vi "OCV Histogram 4309.vi"(8 "Error In":errorcluster, 10 "Results Input":T2={"V ch0 Array"=[], "V ch1 Array"=[], "V ch2 Array"=[], "V ch3 Array"=[], "V ch4 Array"=[], "Elapsed Time (ms)"=11164, "DMM Fault Array"=[]}) -> (0 "Error Out":errorcluster, 1 "mean values of channels":dbl[](array[numeric])=[-6.648192609520545e-06, -2.6579412172609335e-06, 5.730660716698524e-06, 9.480335334891014e-06, -2.6031729589807576e-07] format="%#_7p", 2 "std dev":dbl=4.593584714427233e-07 format="%.3p", 3 "range":dbl=1.8604783993401584e-06 format="%.3p", 4 "Results Output":T1={"ch3 range"=1.5284304409643419e-06, "ch3 std dev"=3.7432297421944963e-07, "ch3 mean"=9.480335334891014e-06, "Histogram Graph ch3"={"X Values"=[8.804122636382775e-06, 8.956965680479209e-06, 9.109808724575643e-06, 9.262651768672077e-06, 9.415494812768511e-06, 9.568337856864946e-06, 9.72118090096138e-06, 9.874023945057814e-06, 1.0026866989154248e-05, 1.0179710033250682e-05], "Histogram: h(x)"=[2, 4, 3, 7, 5, 3, 7, 6, 1, 2]}, "ch2 range"=1.9041594218219493e-06, "ch2 std dev"=4.1579103732429095e-07, "ch2 mean"=5.730660716698524e-06, "Histogram Graph ch2"={"X Values"=[4.8417078226500296e-06, 5.032123764832224e-06, 5.222539707014419e-06, 5.412955649196613e-06, 5.603371591378808e-06, 5.7937875335610025e-06, 5.984203475743197e-06, 6.174619417925392e-06, 6.365035360107586e-06, 6.555451302289781e-06], "Histogram: h(x)"=[2, 2, 4, 3, 5, 8, 9, 5, 1, 1]}, "ch1 range"=1.7442902903444177e-06, "ch1 std dev"=4.468204660544414e-07, "ch1 mean"=-2.6579412172609335e-06, "Histogram Graph ch1"={"X Values"=[-3.3982864936427982e-06, -3.2238574646083565e-06, -3.0494284355739147e-06, -2.874999406539473e-06, -2.700570377505031e-06, -2.5261413484705894e-06, -2.3517123194361476e-06, -2.177283290401706e-06, -2.002854261367264e-06, -1.8284252323328223e-06], "Histogram: h(x)"=[4, 3, 5, 1, 6, 8, 4, 5, 3, 1]}, "ch0 range"=1.9838415017287296e-06, "ch0 std dev"=5.022029434534627e-07, "ch0 mean"=-6.648192609520545e-06, "Histogram Graph ch0"={"X Values"=[-7.4214795585101575e-06, -7.223095408337285e-06, -7.024711258164412e-06, -6.82632710799154e-06, -6.627942957818667e-06, -6.4295588076457944e-06, -6.231174657472922e-06, -6.032790507300049e-06, -5.8344063571271766e-06, -5.636022206954304e-06], "Histogram: h(x)"=[5, 3, 4, 6, 4, 8, 4, 1, 4, 1]}, "Waveform Chart ch1"=[-2.622437675041801e-06, -2.1054414953660847e-06, -2.3277676624794484e-06, -2.558376653803712e-06, -2.2236999675494533e-06, -2.589016451053761e-06, -2.6354278960691e-06, -2.7367192087189563e-06, -2.424017879995447e-06, -3.0489161443253215e-06, -3.1442148467963687e-06, -2.4032855210096374e-06, -2.569647882839888e-06, -2.4698150005498013e-06, -3.0781658817195746e-06, -2.377010372332436e-06, -2.0435595699758798e-06, -2.106839167327596e-06, -1.7412107178156014e-06, -3.2480049993772076e-06, -1.9805074376907754e-06, -2.5608807141114243e-06, -2.18054640635336e-06, -3.099457174386434e-06, -3.102303246629032e-06, -3.2920758007788295e-06, -3.3778499352142414e-06, -3.3187560901861313e-06, -3.484840052811922e-06, -3.485501008160019e-06, -2.8728971850629594e-06, -2.6623123946996634e-06, -2.187546597757112e-06, -2.5467930720162336e-06, -2.7862697099761513e-06, -2.528638777412977e-06, -2.0537236385737207e-06, -2.5329982714180255e-06, -2.7424337661967574e-06, -3.067742416854491e-06], "Waveform Chart ch2"=[5.544446756924017e-06, 5.893818847440082e-06, 5.6959361744068e-06, 6.353655436755351e-06, 6.650659273380882e-06, 6.187390686867271e-06, 6.20360970192913e-06, 5.7770612172558695e-06, 5.816303483036932e-06, 5.681492261411933e-06, 5.92762437831725e-06, 6.190843181120228e-06, 5.928079790707314e-06, 6.068116911256402e-06, 6.161619546592655e-06, 5.5543262999422065e-06, 6.17040032539053e-06, 5.4655577958543896e-06, 5.76704970728763e-06, 6.0194055222271105e-06, 5.783390336812049e-06, 5.768011867723238e-06, 6.0153044120154e-06, 6.001437704705948e-06, 5.911709913790112e-06, 5.830095407868431e-06, 5.25398022881523e-06, 5.15697143423068e-06, 4.826305970962092e-06, 5.462550730311096e-06, 5.059430867978049e-06, 5.682513029845579e-06, 5.851683523904261e-06, 5.099226732675129e-06, 5.2309820281174504e-06, 5.22374278950658e-06, 5.829274618675769e-06, 4.746499851558932e-06, 5.396447289671177e-06, 6.039472630669777e-06], "Waveform Chart ch0"=[-6.482741875349764e-06, -6.609674165618734e-06, -6.233203080218623e-06, -6.613210951394088e-06, -5.909245924550351e-06, -6.1328996888307884e-06, -6.358200673203053e-06, -6.870973185430456e-06, -6.243427483099904e-06, -5.953840097279857e-06, -6.577614794730629e-06, -5.768388563769013e-06, -5.889962020259323e-06, -5.91212430154465e-06, -6.419565311385181e-06, -6.50829315132552e-06, -5.536830131867864e-06, -6.271011369459595e-06, -6.937542782195293e-06, -7.44168991871554e-06, -6.8984467501811205e-06, -7.4441074466820366e-06, -6.884514522294152e-06, -7.229455884586274e-06, -7.204633996616539e-06, -7.520671633596594e-06, -7.348344858091178e-06, -7.026224856705287e-06, -6.4957495291395714e-06, -6.9697185324009035e-06, -6.64170832689038e-06, -6.516226556717238e-06, -6.80187883727134e-06, -7.473746530800666e-06, -6.8019074543289836e-06, -6.421730747707948e-06, -6.915517716049444e-06, -7.233306065769019e-06, -6.9335647318597554e-06, -6.495809932905111e-06], "Waveform Chart ch3"=[9.329772359568193e-06, 9.772186603754015e-06, 9.974785258468733e-06, 1.02561315552989e-05, 9.495402230894659e-06, 9.736598828932665e-06, 9.898850155608759e-06, 1.0197036488504313e-05, 9.305987891150035e-06, 9.316802834906767e-06, 9.746712874470878e-06, 9.737416581604666e-06, 9.867514527065477e-06, 9.509080464808271e-06, 9.481845866845764e-06, 9.70755176396829e-06, 8.885838770613302e-06, 9.475699672125386e-06, 9.258180372816345e-06, 9.834891872602234e-06, 9.402243918552161e-06, 9.713205786936326e-06, 9.876491292911543e-06, 9.871789580104262e-06, 9.650930388911628e-06, 9.41118365911455e-06, 9.575353492249282e-06, 9.196921234035763e-06, 9.15123272945548e-06, 8.949563027841687e-06, 9.474861956745276e-06, 8.825224921180636e-06, 8.727701114334558e-06, 9.16860173648142e-06, 8.905227736485157e-06, 9.144446889757383e-06, 8.885482293855075e-06, 9.859395612279415e-06, 9.32444154185109e-06, 9.310827508550253e-06]} {"ch3 range" format="%#_6p"; "ch3 std dev" format="%#.3p"; "ch3 mean" format="%#.6p"; "ch2 range" format="%#_6p"; "ch2 std dev" format="%#.3p"; "ch2 mean" format="%#.6p"; "ch1 range" format="%#_6p"; "ch1 std dev" format="%#.3p"; "ch1 mean" format="%#.6p"; "ch0 range" format="%#_6p"; "ch0 std dev" format="%#.3p"; "ch0 mean" format="%#.6p"}, 5 "Elapsed Time (ms)":u32)   [LabVIEW 2019]
uses:
  OCVResults.ctl
  Chart_Graph_Mean_Range_StdDev.ctl
  <vilib>/Analysis/baseanly.llb/Mean (DBL).vi
  <vilib>/Analysis/NI_AALBase.lvlib
  <vilib>/gmath/NI_Gmath.lvlib
panel:
  in  "Results Cluster":T1={"ch3 range"=1.5284304409643419e-06, "ch3 std dev"=3.7432297421944963e-07, "ch3 mean"=9.480335334891014e-06, "Histogram Graph ch3"={"X Values"=[8.804122636382775e-06, 8.956965680479209e-06, 9.109808724575643e-06, 9.262651768672077e-06, 9.415494812768511e-06, 9.568337856864946e-06, 9.72118090096138e-06, 9.874023945057814e-06, 1.0026866989154248e-05, 1.0179710033250682e-05], "Histogram: h(x)"=[2, 4, 3, 7, 5, 3, 7, 6, 1, 2]}, "ch2 range"=1.9041594218219493e-06, "ch2 std dev"=4.1579103732429095e-07, "ch2 mean"=5.730660716698524e-06, "Histogram Graph ch2"={"X Values"=[4.8417078226500296e-06, 5.032123764832224e-06, 5.222539707014419e-06, 5.412955649196613e-06, 5.603371591378808e-06, 5.7937875335610025e-06, 5.984203475743197e-06, 6.174619417925392e-06, 6.365035360107586e-06, 6.555451302289781e-06], "Histogram: h(x)"=[2, 2, 4, 3, 5, 8, 9, 5, 1, 1]}, "ch1 range"=1.7442902903444177e-06, "ch1 std dev"=4.468204660544414e-07, "ch1 mean"=-2.6579412172609335e-06, "Histogram Graph ch1"={"X Values"=[-3.3982864936427982e-06, -3.2238574646083565e-06, -3.0494284355739147e-06, -2.874999406539473e-06, -2.700570377505031e-06, -2.5261413484705894e-06, -2.3517123194361476e-06, -2.177283290401706e-06, -2.002854261367264e-06, -1.8284252323328223e-06], "Histogram: h(x)"=[4, 3, 5, 1, 6, 8, 4, 5, 3, 1]}, "ch0 range"=1.9838415017287296e-06, "ch0 std dev"=5.022029434534627e-07, "ch0 mean"=-6.648192609520545e-06, "Histogram Graph ch0"={"X Values"=[-7.4214795585101575e-06, -7.223095408337285e-06, -7.024711258164412e-06, -6.82632710799154e-06, -6.627942957818667e-06, -6.4295588076457944e-06, -6.231174657472922e-06, -6.032790507300049e-06, -5.8344063571271766e-06, -5.636022206954304e-06], "Histogram: h(x)"=[5, 3, 4, 6, 4, 8, 4, 1, 4, 1]}, "Waveform Chart ch1"=[-2.622437675041801e-06, -2.1054414953660847e-06, -2.3277676624794484e-06, -2.558376653803712e-06, -2.2236999675494533e-06, -2.589016451053761e-06, -2.6354278960691e-06, -2.7367192087189563e-06, -2.424017879995447e-06, -3.0489161443253215e-06, -3.1442148467963687e-06, -2.4032855210096374e-06, -2.569647882839888e-06, -2.4698150005498013e-06, -3.0781658817195746e-06, -2.377010372332436e-06, -2.0435595699758798e-06, -2.106839167327596e-06, -1.7412107178156014e-06, -3.2480049993772076e-06, -1.9805074376907754e-06, -2.5608807141114243e-06, -2.18054640635336e-06, -3.099457174386434e-06, -3.102303246629032e-06, -3.2920758007788295e-06, -3.3778499352142414e-06, -3.3187560901861313e-06, -3.484840052811922e-06, -3.485501008160019e-06, -2.8728971850629594e-06, -2.6623123946996634e-06, -2.187546597757112e-06, -2.5467930720162336e-06, -2.7862697099761513e-06, -2.528638777412977e-06, -2.0537236385737207e-06, -2.5329982714180255e-06, -2.7424337661967574e-06, -3.067742416854491e-06], "Waveform Chart ch2"=[5.544446756924017e-06, 5.893818847440082e-06, 5.6959361744068e-06, 6.353655436755351e-06, 6.650659273380882e-06, 6.187390686867271e-06, 6.20360970192913e-06, 5.7770612172558695e-06, 5.816303483036932e-06, 5.681492261411933e-06, 5.92762437831725e-06, 6.190843181120228e-06, 5.928079790707314e-06, 6.068116911256402e-06, 6.161619546592655e-06, 5.5543262999422065e-06, 6.17040032539053e-06, 5.4655577958543896e-06, 5.76704970728763e-06, 6.0194055222271105e-06, 5.783390336812049e-06, 5.768011867723238e-06, 6.0153044120154e-06, 6.001437704705948e-06, 5.911709913790112e-06, 5.830095407868431e-06, 5.25398022881523e-06, 5.15697143423068e-06, 4.826305970962092e-06, 5.462550730311096e-06, 5.059430867978049e-06, 5.682513029845579e-06, 5.851683523904261e-06, 5.099226732675129e-06, 5.2309820281174504e-06, 5.22374278950658e-06, 5.829274618675769e-06, 4.746499851558932e-06, 5.396447289671177e-06, 6.039472630669777e-06], "Waveform Chart ch0"=[-6.482741875349764e-06, -6.609674165618734e-06, -6.233203080218623e-06, -6.613210951394088e-06, -5.909245924550351e-06, -6.1328996888307884e-06, -6.358200673203053e-06, -6.870973185430456e-06, -6.243427483099904e-06, -5.953840097279857e-06, -6.577614794730629e-06, -5.768388563769013e-06, -5.889962020259323e-06, -5.91212430154465e-06, -6.419565311385181e-06, -6.50829315132552e-06, -5.536830131867864e-06, -6.271011369459595e-06, -6.937542782195293e-06, -7.44168991871554e-06, -6.8984467501811205e-06, -7.4441074466820366e-06, -6.884514522294152e-06, -7.229455884586274e-06, -7.204633996616539e-06, -7.520671633596594e-06, -7.348344858091178e-06, -7.026224856705287e-06, -6.4957495291395714e-06, -6.9697185324009035e-06, -6.64170832689038e-06, -6.516226556717238e-06, -6.80187883727134e-06, -7.473746530800666e-06, -6.8019074543289836e-06, -6.421730747707948e-06, -6.915517716049444e-06, -7.233306065769019e-06, -6.9335647318597554e-06, -6.495809932905111e-06], "Waveform Chart ch3"=[9.329772359568193e-06, 9.772186603754015e-06, 9.974785258468733e-06, 1.02561315552989e-05, 9.495402230894659e-06, 9.736598828932665e-06, 9.898850155608759e-06, 1.0197036488504313e-05, 9.305987891150035e-06, 9.316802834906767e-06, 9.746712874470878e-06, 9.737416581604666e-06, 9.867514527065477e-06, 9.509080464808271e-06, 9.481845866845764e-06, 9.70755176396829e-06, 8.885838770613302e-06, 9.475699672125386e-06, 9.258180372816345e-06, 9.834891872602234e-06, 9.402243918552161e-06, 9.713205786936326e-06, 9.876491292911543e-06, 9.871789580104262e-06, 9.650930388911628e-06, 9.41118365911455e-06, 9.575353492249282e-06, 9.196921234035763e-06, 9.15123272945548e-06, 8.949563027841687e-06, 9.474861956745276e-06, 8.825224921180636e-06, 8.727701114334558e-06, 9.16860173648142e-06, 8.905227736485157e-06, 9.144446889757383e-06, 8.885482293855075e-06, 9.859395612279415e-06, 9.32444154185109e-06, 9.310827508550253e-06]} {"ch3 range" format="%#_6p"; "ch3 std dev" format="%#.3p"; "ch3 mean" format="%#.6p"; "ch2 range" format="%#_6p"; "ch2 std dev" format="%#.3p"; "ch2 mean" format="%#.6p"; "ch1 range" format="%#_6p"; "ch1 std dev" format="%#.3p"; "ch1 mean" format="%#.6p"; "ch0 range" format="%#_6p"; "ch0 std dev" format="%#.3p"; "ch0 mean" format="%#.6p"}
  in  "4309 500 Hz":T2={"V ch0 Array"=[], "V ch1 Array"=[], "V ch2 Array"=[], "V ch3 Array"=[], "V ch4 Array"=[], "Elapsed Time (ms)"=11164, "DMM Fault Array"=[]}
  in  "4309 200 Hz":T2={"V ch0 Array"=[], "V ch1 Array"=[], "V ch2 Array"=[], "V ch3 Array"=[], "V ch4 Array"=[], "Elapsed Time (ms)"=11164, "DMM Fault Array"=[]}
  in  "4309 100 Hz":T2={"V ch0 Array"=[], "V ch1 Array"=[], "V ch2 Array"=[], "V ch3 Array"=[], "V ch4 Array"=[], "Elapsed Time (ms)"=11164, "DMM Fault Array"=[]}
  in  "4309 10 Hz":T2={"V ch0 Array"=[], "V ch1 Array"=[], "V ch2 Array"=[], "V ch3 Array"=[], "V ch4 Array"=[], "Elapsed Time (ms)"=11164, "DMM Fault Array"=[]}
  in  "4309 12 Hz":T2={"V ch0 Array"=[], "V ch1 Array"=[], "V ch2 Array"=[], "V ch3 Array"=[], "V ch4 Array"=[], "Elapsed Time (ms)"=11164, "DMM Fault Array"=[]}
  in  "4309 15 Hz":T2={"V ch0 Array"=[], "V ch1 Array"=[], "V ch2 Array"=[], "V ch3 Array"=[], "V ch4 Array"=[], "Elapsed Time (ms)"=11164, "DMM Fault Array"=[]}
  in  "4309 20 Hz":T2={"V ch0 Array"=[], "V ch1 Array"=[], "V ch2 Array"=[], "V ch3 Array"=[], "V ch4 Array"=[], "Elapsed Time (ms)"=11164, "DMM Fault Array"=[]}
  in  "4309 30 Hz":T2={"V ch0 Array"=[], "V ch1 Array"=[], "V ch2 Array"=[], "V ch3 Array"=[], "V ch4 Array"=[], "Elapsed Time (ms)"=11164, "DMM Fault Array"=[]}
  in  "4309 60 Hz":T2={"V ch0 Array"=[], "V ch1 Array"=[], "V ch2 Array"=[], "V ch3 Array"=[], "V ch4 Array"=[], "Elapsed Time (ms)"=11164, "DMM Fault Array"=[]}
  out "ch3 range":dbl=1.5284304409643419e-06 format="%#_6p"
  out "ch3 std dev":dbl=3.7432297421944963e-07 format="%#.3p"
  out "ch3 mean":dbl=9.480335334891014e-06 format="%#.6p"
  out "Histogram Graph ch3":T3(graph)={"X Values"=[8.804122636382775e-06, 8.956965680479209e-06, 9.109808724575643e-06, 9.262651768672077e-06, 9.415494812768511e-06, 9.568337856864946e-06, 9.72118090096138e-06, 9.874023945057814e-06, 1.0026866989154248e-05, 1.0179710033250682e-05], "Histogram: h(x)"=[2, 4, 3, 7, 5, 3, 7, 6, 1, 2]}
  out "ch2 range":dbl=1.9041594218219493e-06 format="%#_6p"
  out "ch2 std dev":dbl=4.1579103732429095e-07 format="%#.3p"
  out "ch2 mean":dbl=5.730660716698524e-06 format="%#.6p"
  out "Histogram Graph ch2":T3(graph)={"X Values"=[4.8417078226500296e-06, 5.032123764832224e-06, 5.222539707014419e-06, 5.412955649196613e-06, 5.603371591378808e-06, 5.7937875335610025e-06, 5.984203475743197e-06, 6.174619417925392e-06, 6.365035360107586e-06, 6.555451302289781e-06], "Histogram: h(x)"=[2, 2, 4, 3, 5, 8, 9, 5, 1, 1]}
  out "ch1 range":dbl=1.7442902903444177e-06 format="%#_6p"
  out "ch1 std dev":dbl=4.468204660544414e-07 format="%#.3p"
  out "ch1 mean":dbl=-2.6579412172609335e-06 format="%#.6p"
  out "Histogram Graph ch1":T3(graph)={"X Values"=[-3.3982864936427982e-06, -3.2238574646083565e-06, -3.0494284355739147e-06, -2.874999406539473e-06, -2.700570377505031e-06, -2.5261413484705894e-06, -2.3517123194361476e-06, -2.177283290401706e-06, -2.002854261367264e-06, -1.8284252323328223e-06], "Histogram: h(x)"=[4, 3, 5, 1, 6, 8, 4, 5, 3, 1]}
  out "ch0 range":dbl=1.9838415017287296e-06 format="%#_6p"
  out "ch0 std dev":dbl=5.022029434534627e-07 format="%#.3p"
  out "ch0 mean":dbl=-6.648192609520545e-06 format="%#.6p"
  out "Histogram Graph ch0":T3(graph)={"X Values"=[-7.4214795585101575e-06, -7.223095408337285e-06, -7.024711258164412e-06, -6.82632710799154e-06, -6.627942957818667e-06, -6.4295588076457944e-06, -6.231174657472922e-06, -6.032790507300049e-06, -5.8344063571271766e-06, -5.636022206954304e-06], "Histogram: h(x)"=[5, 3, 4, 6, 4, 8, 4, 1, 4, 1]}
  out "Waveform Chart ch1":dbl[](graph)=[-2.622437675041801e-06, -2.1054414953660847e-06, -2.3277676624794484e-06, -2.558376653803712e-06, -2.2236999675494533e-06, -2.589016451053761e-06, -2.6354278960691e-06, -2.7367192087189563e-06, -2.424017879995447e-06, -3.0489161443253215e-06, -3.1442148467963687e-06, -2.4032855210096374e-06, -2.569647882839888e-06, -2.4698150005498013e-06, -3.0781658817195746e-06, -2.377010372332436e-06, -2.0435595699758798e-06, -2.106839167327596e-06, -1.7412107178156014e-06, -3.2480049993772076e-06, -1.9805074376907754e-06, -2.5608807141114243e-06, -2.18054640635336e-06, -3.099457174386434e-06, -3.102303246629032e-06, -3.2920758007788295e-06, -3.3778499352142414e-06, -3.3187560901861313e-06, -3.484840052811922e-06, -3.485501008160019e-06, -2.8728971850629594e-06, -2.6623123946996634e-06, -2.187546597757112e-06, -2.5467930720162336e-06, -2.7862697099761513e-06, -2.528638777412977e-06, -2.0537236385737207e-06, -2.5329982714180255e-06, -2.7424337661967574e-06, -3.067742416854491e-06]
  out "Waveform Chart ch2":dbl[](graph)=[5.544446756924017e-06, 5.893818847440082e-06, 5.6959361744068e-06, 6.353655436755351e-06, 6.650659273380882e-06, 6.187390686867271e-06, 6.20360970192913e-06, 5.7770612172558695e-06, 5.816303483036932e-06, 5.681492261411933e-06, 5.92762437831725e-06, 6.190843181120228e-06, 5.928079790707314e-06, 6.068116911256402e-06, 6.161619546592655e-06, 5.5543262999422065e-06, 6.17040032539053e-06, 5.4655577958543896e-06, 5.76704970728763e-06, 6.0194055222271105e-06, 5.783390336812049e-06, 5.768011867723238e-06, 6.0153044120154e-06, 6.001437704705948e-06, 5.911709913790112e-06, 5.830095407868431e-06, 5.25398022881523e-06, 5.15697143423068e-06, 4.826305970962092e-06, 5.462550730311096e-06, 5.059430867978049e-06, 5.682513029845579e-06, 5.851683523904261e-06, 5.099226732675129e-06, 5.2309820281174504e-06, 5.22374278950658e-06, 5.829274618675769e-06, 4.746499851558932e-06, 5.396447289671177e-06, 6.039472630669777e-06]
  out "Waveform Chart ch0":dbl[](graph)=[-6.482741875349764e-06, -6.609674165618734e-06, -6.233203080218623e-06, -6.613210951394088e-06, -5.909245924550351e-06, -6.1328996888307884e-06, -6.358200673203053e-06, -6.870973185430456e-06, -6.243427483099904e-06, -5.953840097279857e-06, -6.577614794730629e-06, -5.768388563769013e-06, -5.889962020259323e-06, -5.91212430154465e-06, -6.419565311385181e-06, -6.50829315132552e-06, -5.536830131867864e-06, -6.271011369459595e-06, -6.937542782195293e-06, -7.44168991871554e-06, -6.8984467501811205e-06, -7.4441074466820366e-06, -6.884514522294152e-06, -7.229455884586274e-06, -7.204633996616539e-06, -7.520671633596594e-06, -7.348344858091178e-06, -7.026224856705287e-06, -6.4957495291395714e-06, -6.9697185324009035e-06, -6.64170832689038e-06, -6.516226556717238e-06, -6.80187883727134e-06, -7.473746530800666e-06, -6.8019074543289836e-06, -6.421730747707948e-06, -6.915517716049444e-06, -7.233306065769019e-06, -6.9335647318597554e-06, -6.495809932905111e-06]
  out "Waveform Chart ch3":dbl[](graph)=[9.329772359568193e-06, 9.772186603754015e-06, 9.974785258468733e-06, 1.02561315552989e-05, 9.495402230894659e-06, 9.736598828932665e-06, 9.898850155608759e-06, 1.0197036488504313e-05, 9.305987891150035e-06, 9.316802834906767e-06, 9.746712874470878e-06, 9.737416581604666e-06, 9.867514527065477e-06, 9.509080464808271e-06, 9.481845866845764e-06, 9.70755176396829e-06, 8.885838770613302e-06, 9.475699672125386e-06, 9.258180372816345e-06, 9.834891872602234e-06, 9.402243918552161e-06, 9.713205786936326e-06, 9.876491292911543e-06, 9.871789580104262e-06, 9.650930388911628e-06, 9.41118365911455e-06, 9.575353492249282e-06, 9.196921234035763e-06, 9.15123272945548e-06, 8.949563027841687e-06, 9.474861956745276e-06, 8.825224921180636e-06, 8.727701114334558e-06, 9.16860173648142e-06, 8.905227736485157e-06, 9.144446889757383e-06, 8.885482293855075e-06, 9.859395612279415e-06, 9.32444154185109e-06, 9.310827508550253e-06]
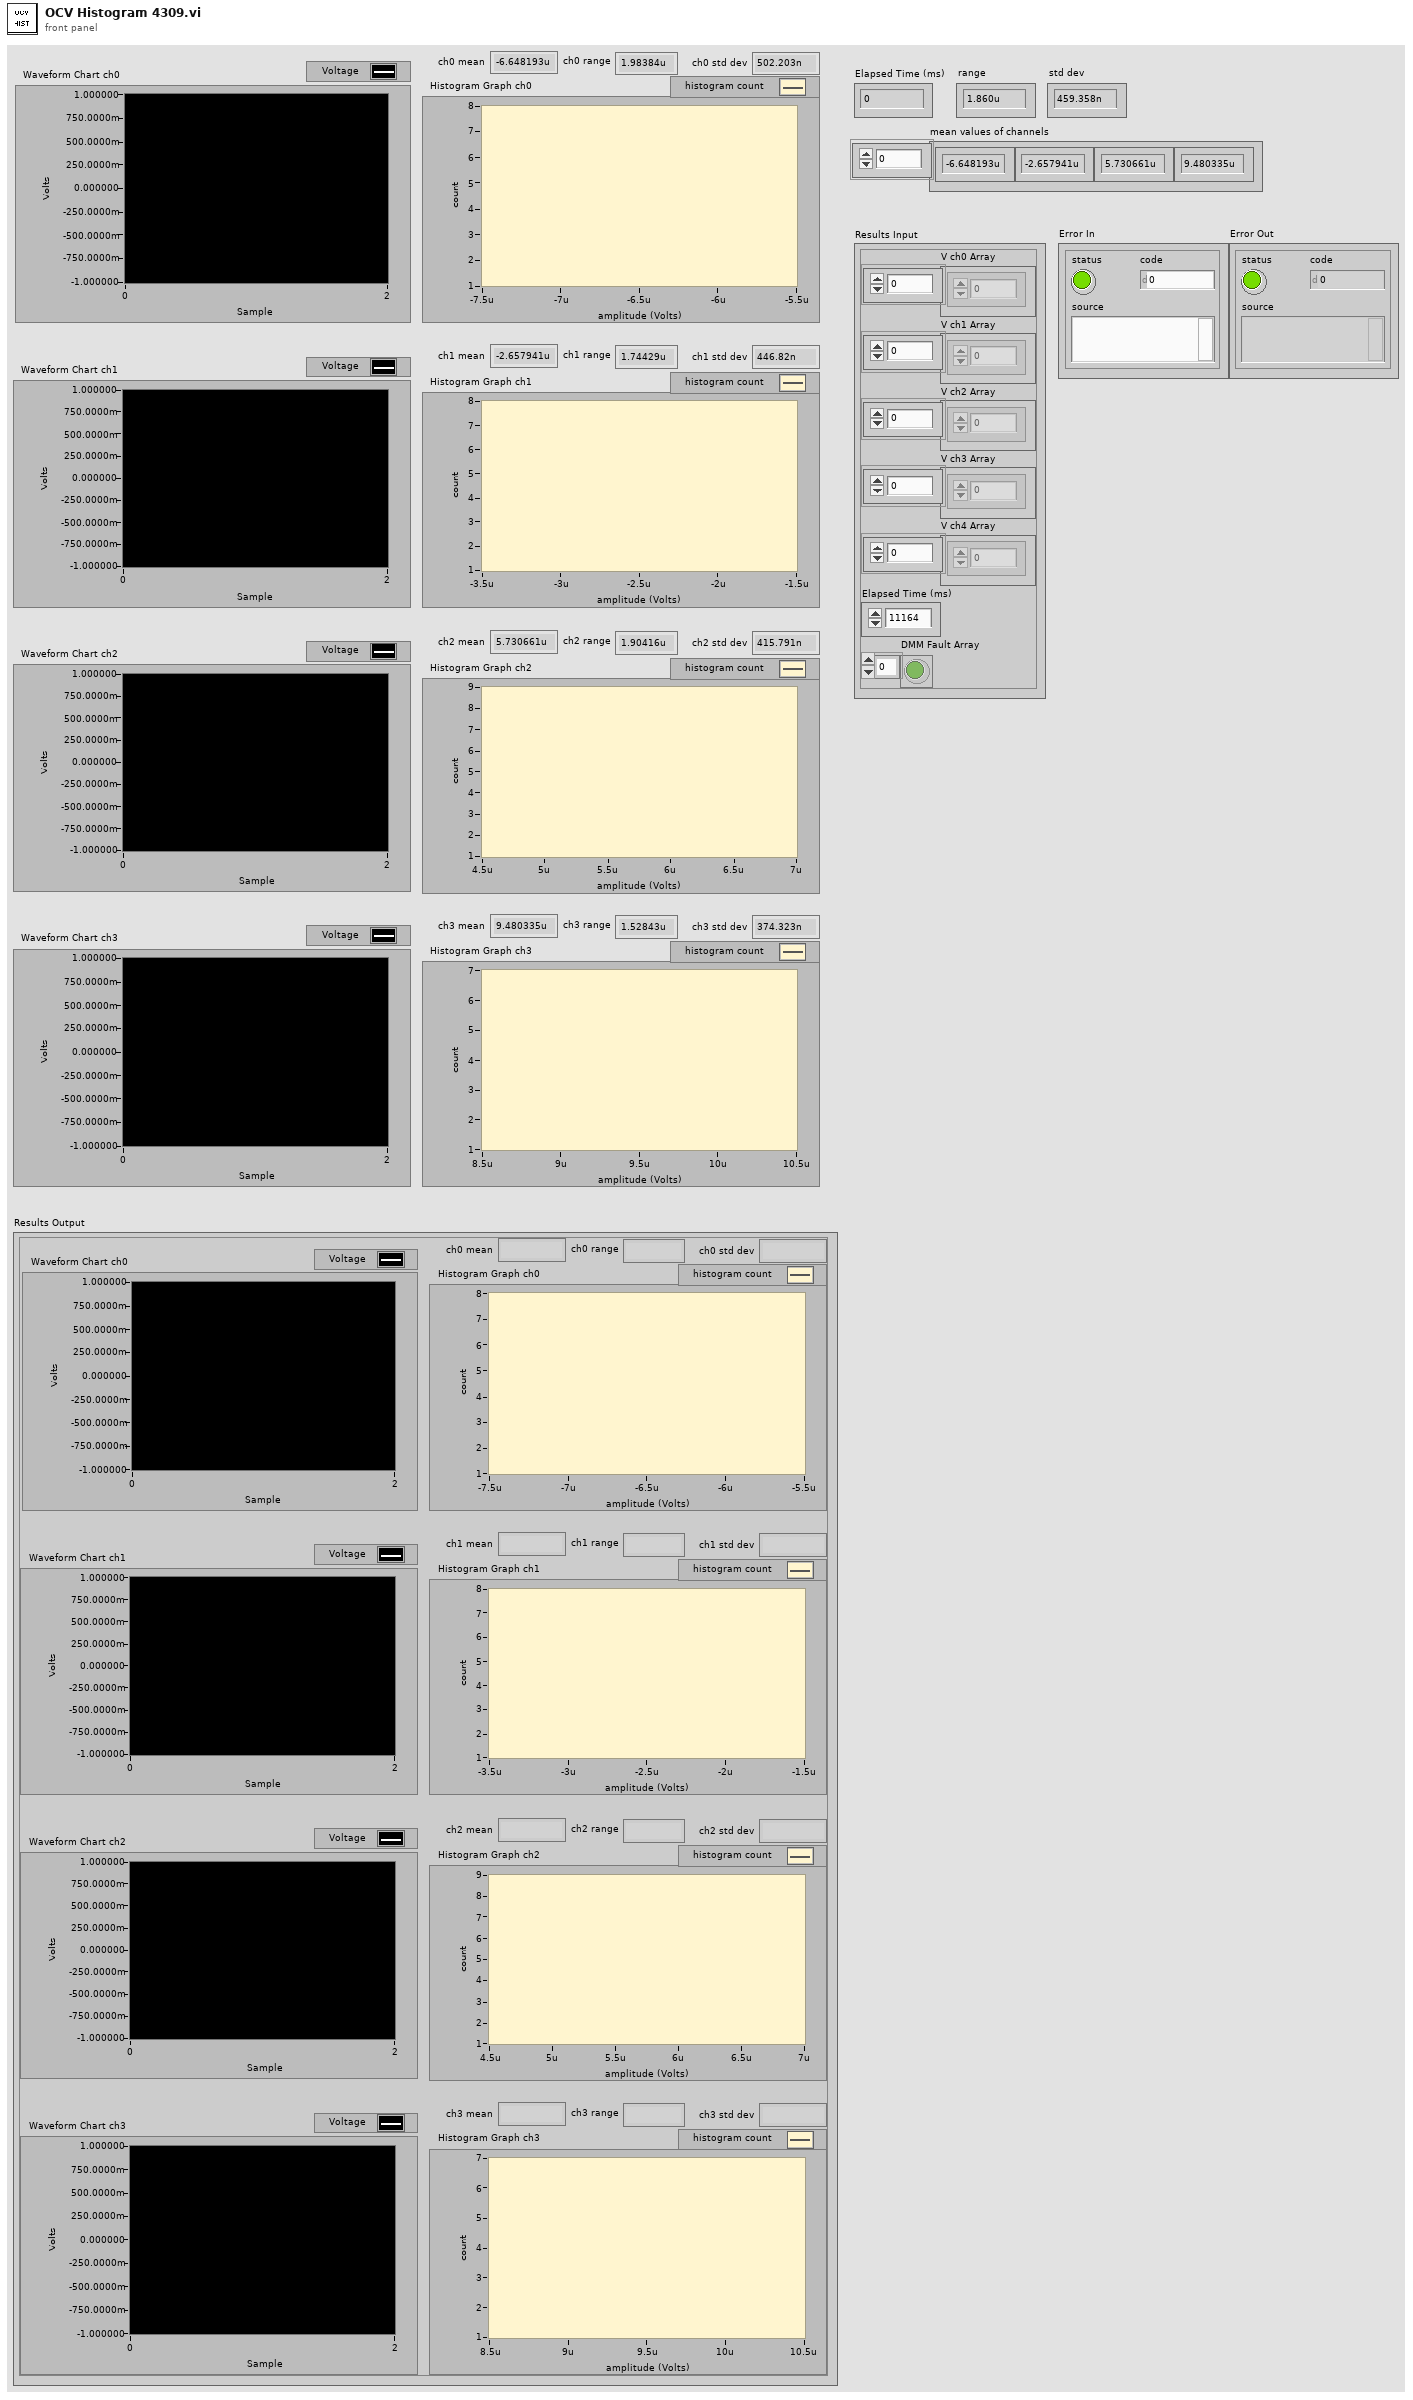
[diagram p1: front panel]
types:
  T1 = typedef "Chart_Graph_Mean_Range_StdDev.ctl" = cluster{"ch3 range":dbl, "ch3 std dev":dbl, "ch3 mean":dbl, "Histogram Graph ch3":cluster{"X Values":dbl[], "Histogram: h(x)":i32[]}, "ch2 range":dbl, "ch2 std dev":dbl, "ch2 mean":dbl, "Histogram Graph ch2":cluster{"X Values":dbl[], "Histogram: h(x)":i32[]}, "ch1 range":dbl, "ch1 std dev":dbl, "ch1 mean":dbl, "Histogram Graph ch1":cluster{"X Values":dbl[], "Histogram: h(x)":i32[]}, "ch0 range":dbl, "ch0 std dev":dbl, "ch0 mean":dbl, "Histogram Graph ch0":cluster{"X Values":dbl[], "Histogram: h(x)":i32[]}, "Waveform Chart ch1":dbl[], "Waveform Chart ch2":dbl[], "Waveform Chart ch0":dbl[], "Waveform Chart ch3":dbl[]}
  T2 = typedef "OCVResults.ctl" = cluster{"V ch0 Array":dbl[], "V ch1 Array":dbl[], "V ch2 Array":dbl[], "V ch3 Array":dbl[], "V ch4 Array":dbl[], "Elapsed Time (ms)":u32, "DMM Fault Array":bool[]}
  T3 = cluster{"X Values":dbl[], "Histogram: h(x)":i32[]}
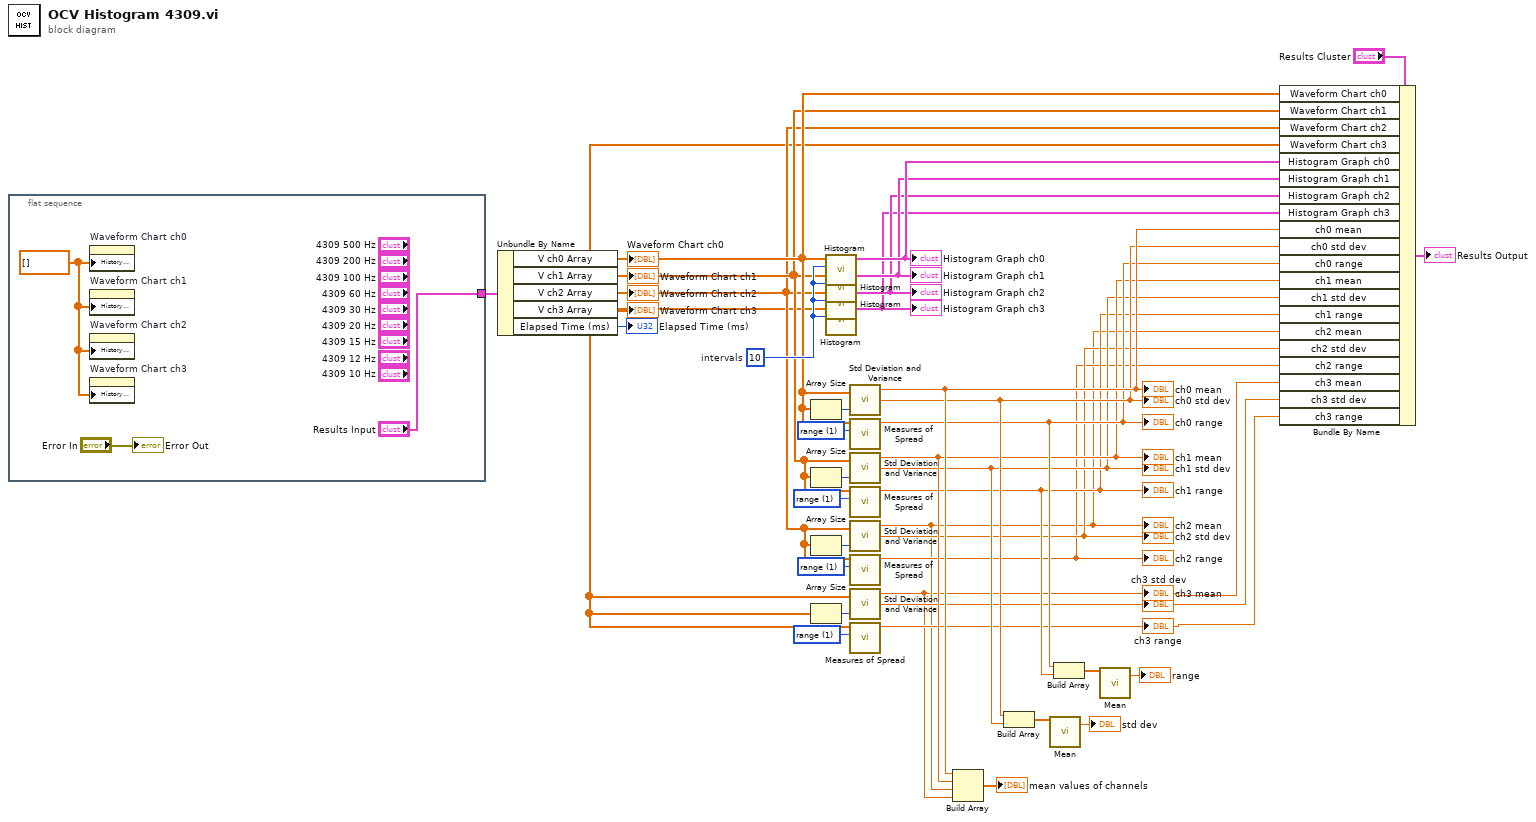
[diagram p0: block diagram]
diagram:
  w30 = 1 items=["standard deviation", "range", "mean absolute deviation", "interquartile range"] ("type")
  w32 = 1 items=["standard deviation", "range", "mean absolute deviation", "interquartile range"] ("type")
  w34 = 1 items=["standard deviation", "range", "mean absolute deviation", "interquartile range"] ("type")
  w36 = 1 items=["standard deviation", "range", "mean absolute deviation", "interquartile range"] ("type")
  w38 = 10  # intervals
  n1 = flat-sequence {
    tunnel: ["Results Input"] -> w24
    frame #0 {
      w41 = dbl[] [] ("History Data")
      n2 = property on="Waveform Chart ch0" class="WFChart (strict)"("History Data"=w41) -> ()  [unwired: 2 in, 2 out]
      n3 = property on="Waveform Chart ch1" class="WFChart (strict)"("History Data"=w41) -> ()  [unwired: 2 in, 2 out]
      n4 = property on="Waveform Chart ch2" class="WFChart (strict)"("History Data"=w41) -> ()  [unwired: 2 in, 2 out]
      n5 = property on="Waveform Chart ch3" class="WFChart (strict)"("History Data"=w41) -> ()  [unwired: 2 in, 2 out]
      "Error Out" <- "Error In"
    }
  }
  n6 = Unbundle By Name(w24) -> ("V ch0 Array"=w21:dbl[], "V ch1 Array"=w20:dbl[], "V ch2 Array"=w19:dbl[], "V ch3 Array"=w18:dbl[], "Elapsed Time (ms)"=→"Elapsed Time (ms)":u32)
  "Waveform Chart ch3" <- w18
  "Waveform Chart ch0" <- w21
  "Waveform Chart ch2" <- w19
  "Waveform Chart ch1" <- w20
  n7 = Array Size(array=w21) -> (size(s)=w37:i32)
  n8 = Array Size(array=w20) -> (size(s)=w35:i32)
  n9 = Array Size(array=w19) -> (size(s)=w33:i32)
  n10 = Array Size(array=w18) -> (size(s)=w31:i32)
  n11 = call <vilib>:"Histogram.vi"("intervals"=w38, "X"=w21) -> ("Histogram Graph"=w17:T3)  [unwired: 6 in, 3 out]
  "Histogram Graph ch0" <- w17
  n12 = call <vilib>:"Histogram.vi"("intervals"=w38, "X"=w20) -> ("Histogram Graph"=w16:T3)  [unwired: 6 in, 3 out]
  "Histogram Graph ch1" <- w16
  n13 = call <vilib>:"Histogram.vi"("intervals"=w38, "X"=w19) -> ("Histogram Graph"=w15:T3)  [unwired: 6 in, 3 out]
  "Histogram Graph ch2" <- w15
  n14 = call <vilib>:"Histogram.vi"("intervals"=w38, "X"=w18) -> ("Histogram Graph"=w14:T3)  [unwired: 6 in, 3 out]
  "Histogram Graph ch3" <- w14
  n15 = call <vilib>:"Std Deviation and Variance.vi"("X"=w21, "Weighting (Sample)"=w37) -> ("mean"=w13:dbl, "standard deviation"=w12:dbl)  [unwired: 1 out]
  "ch0 mean" <- w13
  "ch0 std dev" <- w12
  n16 = call <vilib>:"Measures of Spread.vi"("type"=w36, "x array"=w21) -> ("spread value"=w11:dbl)  [unwired: 8 in, 1 out]
  "ch0 range" <- w11
  n17 = call <vilib>:"Std Deviation and Variance.vi"("X"=w20, "Weighting (Sample)"=w35) -> ("mean"=w10:dbl, "standard deviation"=w9:dbl)  [unwired: 1 out]
  "ch1 mean" <- w10
  "ch1 std dev" <- w9
  n18 = call <vilib>:"Measures of Spread.vi"("type"=w34, "x array"=w20) -> ("spread value"=w8:dbl)  [unwired: 8 in, 1 out]
  "ch1 range" <- w8
  n19 = call <vilib>:"Std Deviation and Variance.vi"("X"=w19, "Weighting (Sample)"=w33) -> ("mean"=w2:dbl, "standard deviation"=w7:dbl)  [unwired: 1 out]
  "ch2 mean" <- w2
  "ch2 std dev" <- w7
  n20 = call <vilib>:"Measures of Spread.vi"("type"=w32, "x array"=w19) -> ("spread value"=w6:dbl)  [unwired: 8 in, 1 out]
  "ch2 range" <- w6
  n21 = call <vilib>:"Std Deviation and Variance.vi"("X"=w18, "Weighting (Sample)"=w31) -> ("mean"=w1:dbl, "standard deviation"=w5:dbl)  [unwired: 1 out]
  "ch3 mean" <- w1
  "ch3 std dev" <- w5
  n22 = call <vilib>:"Measures of Spread.vi"("type"=w30, "x array"=w18) -> ("spread value"=w4:dbl)  [unwired: 8 in, 1 out]
  "ch3 range" <- w4
  n23 = Build Array(w13, w10, w2, w1) -> (→"mean values of channels":dbl[])
  n24 = Build Array(w12, w9) -> (w28:dbl[])
  n25 = call-poly <vilib>:"Mean.vi"("X"=w28) -> ("mean"=→"std dev":dbl)  [unwired: 1 out]
  n26 = Build Array(w11, w8) -> (w26:dbl[])
  n27 = call-poly <vilib>:"Mean.vi"("X"=w26) -> ("mean"=→"range":dbl)  [unwired: 1 out]
  n28 = Bundle By Name(cluster="Results Cluster", "Waveform Chart ch0"=w21, "Waveform Chart ch1"=w20, "Waveform Chart ch2"=w19, "Waveform Chart ch3"=w18, "Histogram Graph ch0"=w17, "Histogram Graph ch1"=w16, "Histogram Graph ch2"=w15, "Histogram Graph ch3"=w14, "ch0 mean"=w13, "ch0 std dev"=w12, "ch0 range"=w11, "ch1 mean"=w10, "ch1 std dev"=w9, "ch1 range"=w8, "ch2 mean"=w2, "ch2 std dev"=w7, "ch2 range"=w6, "ch3 mean"=w1, "ch3 std dev"=w5, "ch3 range"=w4) -> (→"Results Output":T1)
